vi "Test Base Namer with extension no label.vi"   [LabVIEW 2020, in "Namer.Tests.lvclass"]
uses:
  Namer.Tests.lvclass
  Source/Approval Tests/Namer/Namer.lvclass
  Source/Approval Tests/Naming Data/Naming Data.lvclass
  <vilib>/addons/_JKI Toolkits/Caraya/classes/Test/Test.lvclass
  <vilib>/addons/_JKI Toolkits/Caraya/classes/Assert/Assert.lvclass
  <vilib>/addons/_JKI Toolkits/Caraya/classes/Assert/Assert Equal Value and Type_Variant.vi
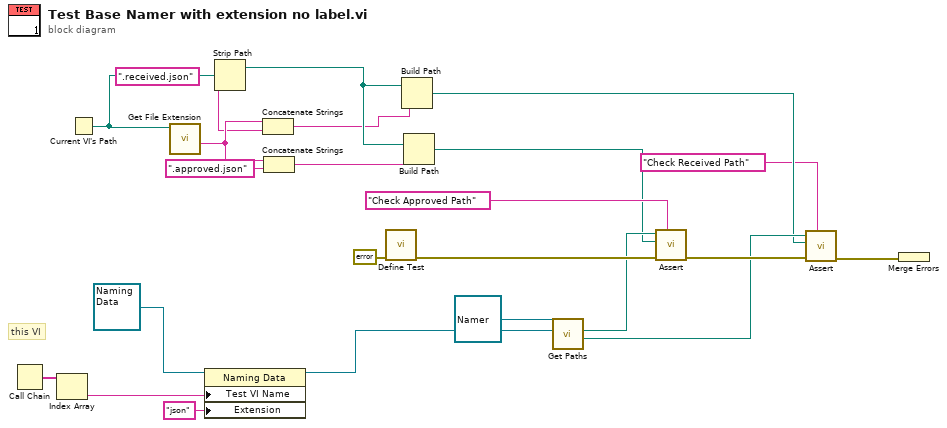
[diagram p0: block diagram]
diagram:
  # "this VI"
  n1 = Call Chain() -> (call chain=w18:string[])
  n2 = Index Array(array=w18) -> (element=w17:string)  [unwired: 1 in]
  n3 = Current VI's Path() -> (path=w11:path)
  n4 = call <vilib>:"Get File Extension.vi"("file"=w11) -> ("filename without extension"=w9:string)  [unwired: 6 in, 4 out]
  n5 = property on="Property Node" class="Naming Data"(reference=refnum<class "Naming Data.lvclass"> refnum ("Naming Data"), "Test VI Name"=w17, "Extension"="json") -> (reference out=w16:refnum<class "Naming Data.lvclass">)  [unwired: 1 in, 1 out]
  n6 = Strip Path(path=w11) -> (stripped path=w10:path)  [unwired: 1 out]
  n7 = Concatenate Strings(w9, ".received.json" ("string")) -> (w6:string)
  n8 = Concatenate Strings(w9, ".approved.json" ("string")) -> (w5:string)
  n9 = call <vilib>:"Define Test.vi"("error in (no error)"=errorcluster {"status"=FALSE, "code"=0, "source"=""}) -> ("error out"=w22:errorcluster)  [unwired: 9 in, 1 out]
  n10 = Build Path(base path=w10, name or relative path=w6) -> (appended path=w4:path)
  n11 = Build Path(base path=w10, name or relative path=w5) -> (appended path=w3:path)
  n12 = call-dynamic "Get Paths.vi"("Naming Data"=w16, "Namer in"=refnum<class "Namer.lvclass"> refnum ("Approval Tests:Namer")) -> ("Received Path"=w12:path, "Approved Path"=w13:path)  [unwired: 6 in, 2 out]
  n13 = call-poly <vilib>:"Assert.vi"("Label"="Check Approved Path" ("Label (VI Title)"), "error in (no error)"=w22, "Actual"=w3, "Expected"=w13) -> ("error out"=w15:errorcluster)  [unwired: 6 in, 1 out]
  n14 = call-poly <vilib>:"Assert.vi"("Label"="Check Received Path" ("Label (VI Title)"), "error in (no error)"=w15, "Actual"=w4, "Expected"=w12) -> ("error out"=w14:errorcluster)  [unwired: 6 in, 1 out]
  n15 = Merge Errors(w14) -> ()  [unwired: 1 out]
